vi "Calc Action Diagram Sizing.vi"(7 "Diagram Ref":refnum<vi>, 11 "Actions In":T1={"Init"=FALSE, "Start"=FALSE, "Run"=TRUE, "Stop"=FALSE, "Close"=FALSE}) -> (3 "Actions":T1={"Init"=FALSE, "Start"=FALSE, "Run"=TRUE, "Stop"=FALSE, "Close"=FALSE}, 5 "Action Diagram Sizing":T2)   [LabVIEW 2022 SP3, in "FlexBlocks Support.lvlib"]
uses:
  FlexBlocks Support.lvlib
  Action Selections.ctl
  Action Diagram Sizing.ctl
panel:
  out "Total Width":i32
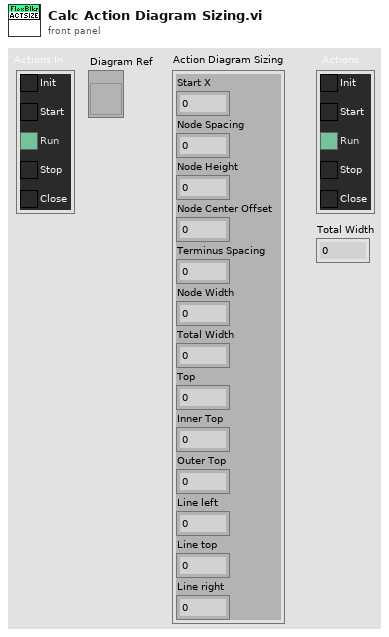
[diagram p1: front panel]
types:
  T1 = typedef "FlexBlocks Support.lvlib/Action Selections.ctl" = cluster{"Init":bool, "Start":bool, "Run":bool, "Stop":bool, "Close":bool}
  T2 = typedef "FlexBlocks Support.lvlib/Action Diagram Sizing.ctl" = cluster{"Start X":i32, "Node Spacing":i32, "Node Height":i32, "Node Center Offset":i32, "Terminus Spacing":i32, "Node Width":i32, "Total Width":i32, "Top":i32, "Inner Top":i32, "Outer Top":i32, "Line left":i32, "Line top":i32, "Line right":i32}
  T3 = typedef "LVBoundsTypeDef.ctl" = cluster{"Width":u32, "Height":u32}
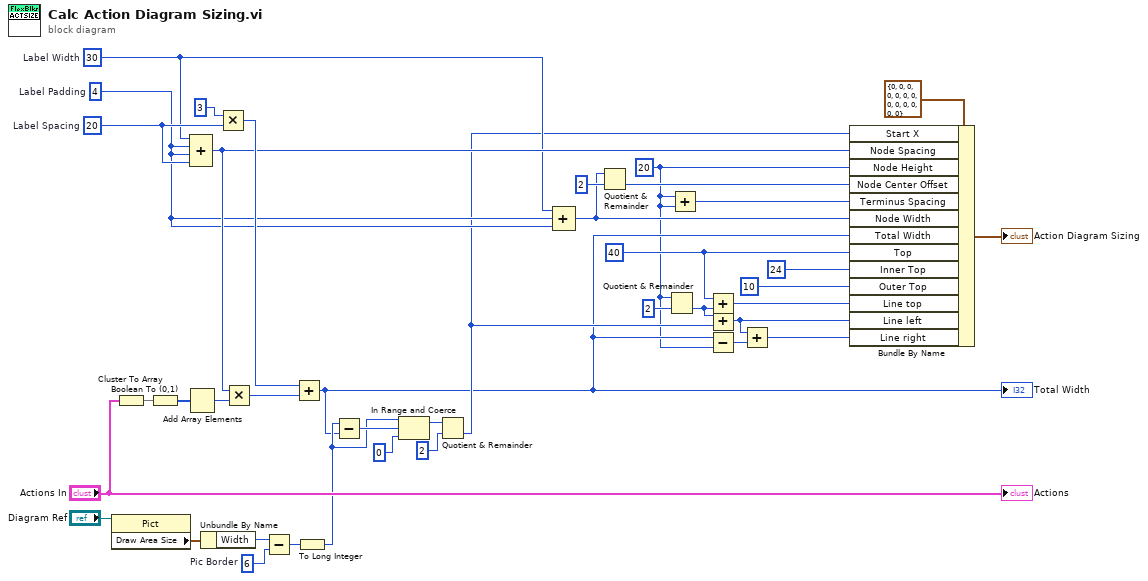
[diagram p0: block diagram]
diagram:
  w9 = 40 ("Top")
  w13 = u32 6  # Pic Border
  w2 = 20 ("Node Height")
  w16 = 4  # Label Padding
  w33 = 20  # Label Spacing
  w17 = 30  # Label Width
  n1 = property class="Pict"(reference="Diagram Ref") -> ("Draw Area Size"=w34:T3)  [unwired: 1 in, 2 out]
  n2 = Cluster To Array(cluster="Actions In") -> (array=w39:bool[])
  n3 = Boolean To (0,1)(Boolean=w39) -> (0, 1=w38:i16[])
  n4 = Add Array Elements(numeric array=w38) -> (sum=w36:i16)
  n5 = Compound Arithmetic op=unknown(w17, w16, w16, w33) -> (w19:i32)
  n6 = Unbundle By Name(w34) -> ("Width"=w29:u32)
  n7 = Multiply(x=3 ("y"), y=w33) -> (x*y=w30:i32)
  n8 = Multiply(x=w19, y=w36) -> (x*y=w31:i32)
  n9 = Subtract(x=w29, y=w13) -> (x-y=w14:u32)
  n10 = Add(x=w30, y=w31) -> (x+y=w5:i32)
  "Total Width" <- w5
  n11 = To Long Integer(number=w14) -> (32bit integer=w20:i32)
  n12 = Subtract(x=w20, y=w5) -> (x-y=w23:i32)
  n13 = In Range and Coerce(upper limit=w20, x=w23, lower limit=0) -> (coerced(x)=w21:i32)  [unwired: 1 out]
  n14 = Quotient & Remainder(x=w21, y=2) -> (floor(x/y)=w7:i32)  [unwired: 1 out]
  n15 = Compound Arithmetic op=unknown(w17, w16, w16) -> (w15:i32)
  n16 = Quotient & Remainder(x=w15, y=2) -> (floor(x/y)=w24:i32)  [unwired: 1 out]
  n17 = Quotient & Remainder(x=w2, y=2) -> (floor(x/y)=w4:i32)  [unwired: 1 out]
  n18 = Add(x=w2, y=w2) -> (x+y=w18:i32)
  n19 = Add(x=w9, y=w4) -> (x+y=w8:i32)
  n20 = Add(x=w4, y=w7) -> (x+y=w6:i32)
  n21 = Subtract(x=w5, y=w2) -> (x-y=w3:i32)
  n22 = Add(x=w6, y=w3) -> (x+y=w1:i32)
  n23 = Bundle By Name(cluster=T2 {"Start X"=0, "Node Spacing"=0, "Node Height"=0, "Node Center Offset"=0, "Terminus Spacing"=0, "Node Width"=0, "Total Width"=0, "Top"=0, "Inner Top"=0, "Outer Top"=0, "Line left"=0, "Line top"=0, "Line right"=0} ("Action Diagram Sizing"), "Start X"=w7, "Node Spacing"=w19, "Node Height"=w2, "Node Center Offset"=w24, "Terminus Spacing"=w18, "Node Width"=w15, "Total Width"=w5, "Top"=w9, "Inner Top"=24, "Outer Top"=10, "Line top"=w8, "Line left"=w6, "Line right"=w1) -> (→"Action Diagram Sizing":T2)
  "Actions" <- "Actions In"
